vi "SubVI.vi"(0 "Points":i32=10) -> (6 "Disorder Pattern 2":dbl[](array[numeric]))   [LabVIEW 2019]
panel:
  in  "Set":bool
  in  "Generate":bool
  out "Disorder Pattern":dbl[](graph)=[1.0078411649904462, 1.0078411649904462, 0.9846991573254764, 0.9846991573254764, 0.9978814600222632, 0.9978814600222632, 0.9723089162683902, 0.9723089162683902, 1.011631648566163, 1.011631648566163]
  in  "App":dbl=0.1
  in  "Step width":dbl=0.2
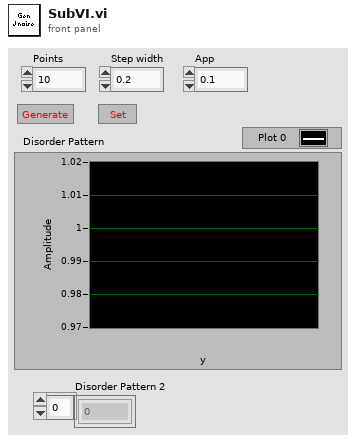
[diagram p1: front panel]
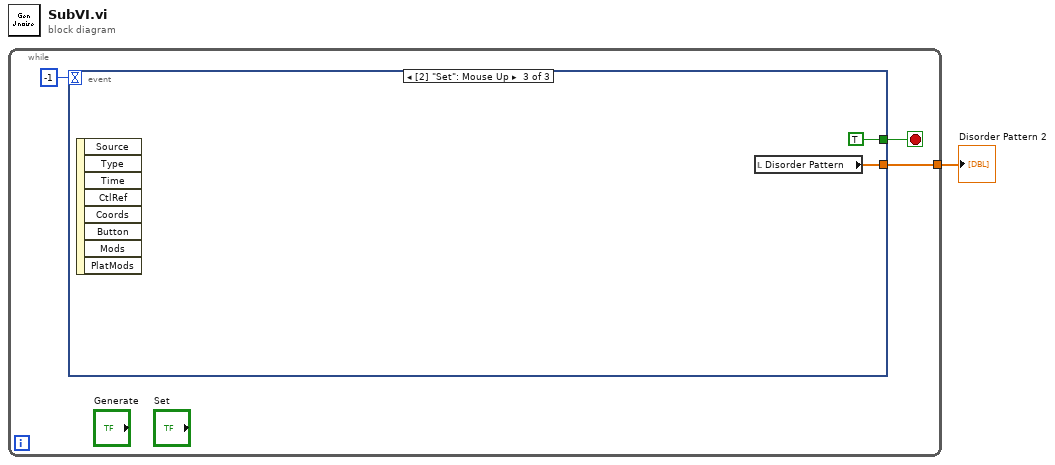
[diagram p0: block diagram]
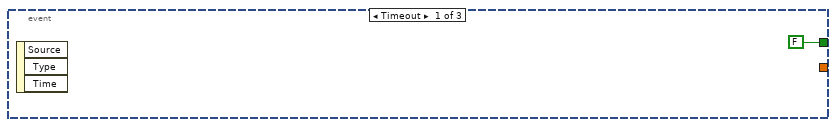
[diagram p2: hidden frame]
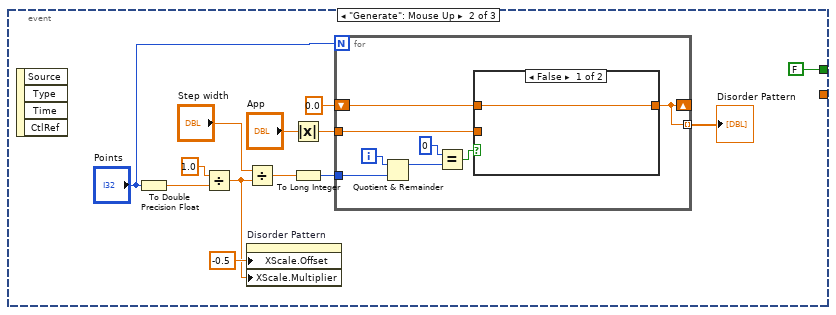
[diagram p3: hidden frame]
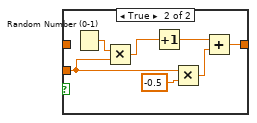
[diagram p4: hidden frame]
diagram:
  n1 = while {
    tunnel: [w2] -> w1
    stop <- w3 stop-if-true
    n2 = event shown="[2] \"Set\": Mouse Up" {
      selector: _ -> [_ _ _]
      dyn-events: _ -> [_ _ _]
      timeout: -1 -> [_ _ _]
      tunnel: [FALSE FALSE TRUE] -> w3
      tunnel: [_ _ w36] -> w2
      event Timeout {
        n3 = event-data() -> ()  [unwired: 1 in, 3 out]
      }
      event "Generate": Mouse Up {
        n4 = event-data() -> ()  [unwired: 1 in, 4 out]
        n5 = To Double Precision Float(number="Points") -> (double precision float=w12:dbl)
        n6 = Divide(x=1.0, y=w12) -> (x/y=w6:dbl)
        n7 = Divide(x="Step width", y=w6) -> (x/y=w14:dbl)
        n8 = property on="Disorder Pattern" class="WFGraph (strict)"("XScale.Offset"=-0.5, "XScale.Multiplier"=w6) -> ()  [unwired: 2 in, 2 out]
        n9 = Absolute Value(x="App") -> (abs(x)=w18:dbl)
        n10 = To Long Integer(number=w14) -> (32bit integer=w16:i32)
        n11 = for {
          N: "Points" -> [_]
          tunnel: w16 -> [w25]
          tunnel: w18 -> [w22]
          shift-right: [w20] -> _
          shift-left: 0.0 -> [w21]
          tunnel: [w20] -> w9 mode=indexing
          i -> [w26]
          n12 = Quotient & Remainder(x=w26, y=w25) -> (x-y*floor(x/y)=w19:i32)  [unwired: 1 out]
          n13 = Equal?(x=0, y=w19) -> (x = y?=w23:bool)
          n14 = case shown="False" w23 {
            tunnel: w22 -> [_ w32]
            tunnel: [w27 w28] -> w20
            tunnel: w21 -> [w27 _]
            frame False {
            }
            frame True {
              n15 = Random Number (0-1)() -> (number: 0 to 1=w34:dbl)
              n16 = Multiply(x=w34, y=w32) -> (x*y=w33:dbl)
              n17 = Increment(x=w33) -> (x+1=w30:dbl)
              n18 = Multiply(x=w32, y=-0.5) -> (x*y=w29:dbl)
              n19 = Add(x=w30, y=w29) -> (x+y=w28:dbl)
            }
          }
        }
        "Disorder Pattern" <- w9
      }
      event "Set": Mouse Up {
        n20 = event-data() -> ()  [unwired: 1 in, 8 out]
        n21 = local read "Disorder Pattern"() -> (w36:dbl[])
      }
    }
  }
  "Disorder Pattern 2" <- w1
